vi "Get Server Address.vi"(8 "error in (no error)":errorcluster, 11 "gRPC Server in":refnum<class "Servicer.lvclass">) -> (0 "error out":errorcluster, 2 "Server Address":string, 3 "gRPC Server out":refnum<class "Servicer.lvclass">)   [LabVIEW 2019, in "gRPC-servicer.lvlib" / "Servicer.lvclass"]
uses:
  Servicer.lvclass
  Servicer.lvclass/Servicer.ctl
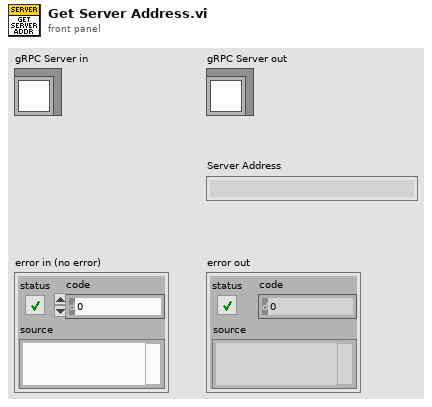
[diagram p1: front panel]
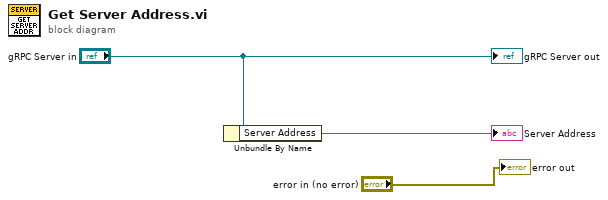
[diagram p0: block diagram]
diagram:
  n1 = Unbundle By Name("gRPC Server in") -> ("Server Address"=→"Server Address":string)
  "gRPC Server out" <- "gRPC Server in"
  "error out" <- "error in (no error)"
